vi "Gateway_GetActiveTunnels.vi"(8 "error in (no error)":errorcluster, 11 "GatewayClass in":refnum<class "GatewayClass.lvclass">) -> (0 "error out":errorcluster, 1 "Local Ports forwarded to SSH":u16[](array[numeric]), 2 "MIDAS Destinations":u16[](array[numeric]), 3 "GatewayClass out":refnum<class "GatewayClass.lvclass">)   [LabVIEW 2018, in "GatewayClass.lvclass"]
uses:
  GatewayClass.lvclass
  GatewayClass.lvclass/GatewayClass.ctl
  DataPacker/Utilities/SSH_TUNNEL.lvclass/SSH_TUNNEL.ctl
  DataPacker/Utilities/SSH_TUNNEL.lvclass
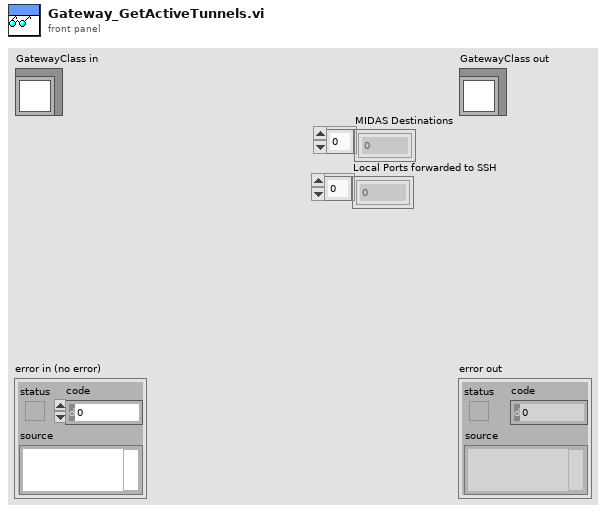
[diagram p1: front panel]
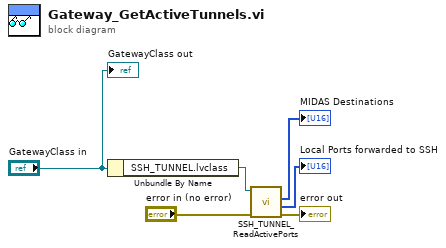
[diagram p0: block diagram]
diagram:
  n1 = Unbundle By Name("GatewayClass in") -> ("SSH_TUNNEL.lvclass"=w3:refnum<class "SSH_TUNNEL.lvclass">)
  n2 = call "SSH_TUNNEL_ReadActivePorts.vi"("error in (no error)"="error in (no error)", "SSH_TUNNEL in"=w3) -> ("error out"=→"error out":errorcluster, "Local Ports forwarded to SSH"=→"Local Ports forwarded to SSH":u16[], "MIDAS Destinations"=→"MIDAS Destinations":u16[])  [unwired: 6 in, 1 out]
  "GatewayClass out" <- "GatewayClass in"
